vi "ExMovCollectIN.vi"() -> ()   [LabVIEW 2010]
panel:
  out "Current Wavelength":string
  in  "Increment Wavelength":dbl=50.0 format="%.2f"
  in  "End Wavelength":dbl=700.0 format="%.2f"
  in  "Start Wavelength":dbl format="%.2f"
  in  "Grating Speed":dbl=2000.0 min=1.0 step=1.0 format="%.2f"
  in  "Grating number":i16=1 min=1 max=100 step=1
  out "Strip":sgl[](graph)
  in  "Temperature":dbl=-10.0 format="%.2f"
  in  "Exposure":dbl min=0.0 step=0.001 format="%.3f"
  in  "stop":bool
  out "error out":errorcluster
  in  "error in (no error)":errorcluster
  # "ExMovCollectIN.vi\nCamera and Spectrometer control of the InSpectrum.  This vi will open both the camera and spectrograph.  It will then move the grating to the Start Wavelength.  Data will then be collected and displayed.  The sequence will be repeated after moving the grating by the Increment Wavelength until the End Wavelength is reached.  At that time, data collection will continue until the STOP button is hit."
  # "NOTES:\nA properly configured spectometer .ini must be present in the LabVIEW folder for spectrograph operation.\n\nConsult the Toolkit documentation for more information on how to configure this file."
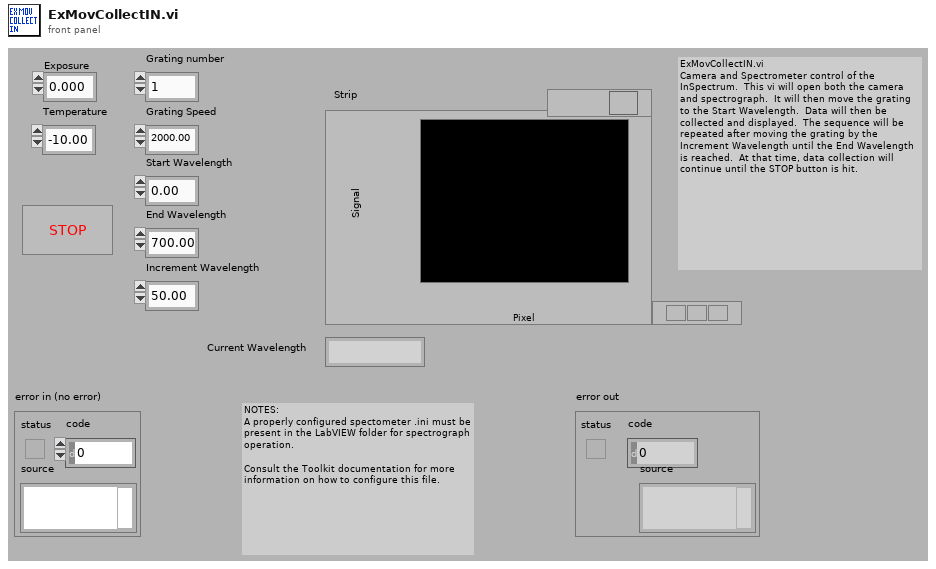
[diagram p1: front panel]
types:
  T1 = cluster{"Camera Handle":u32, "Pulser Handle":u32, "File Handle":u32, "Display Handle":u32, "Image Handle":u32}
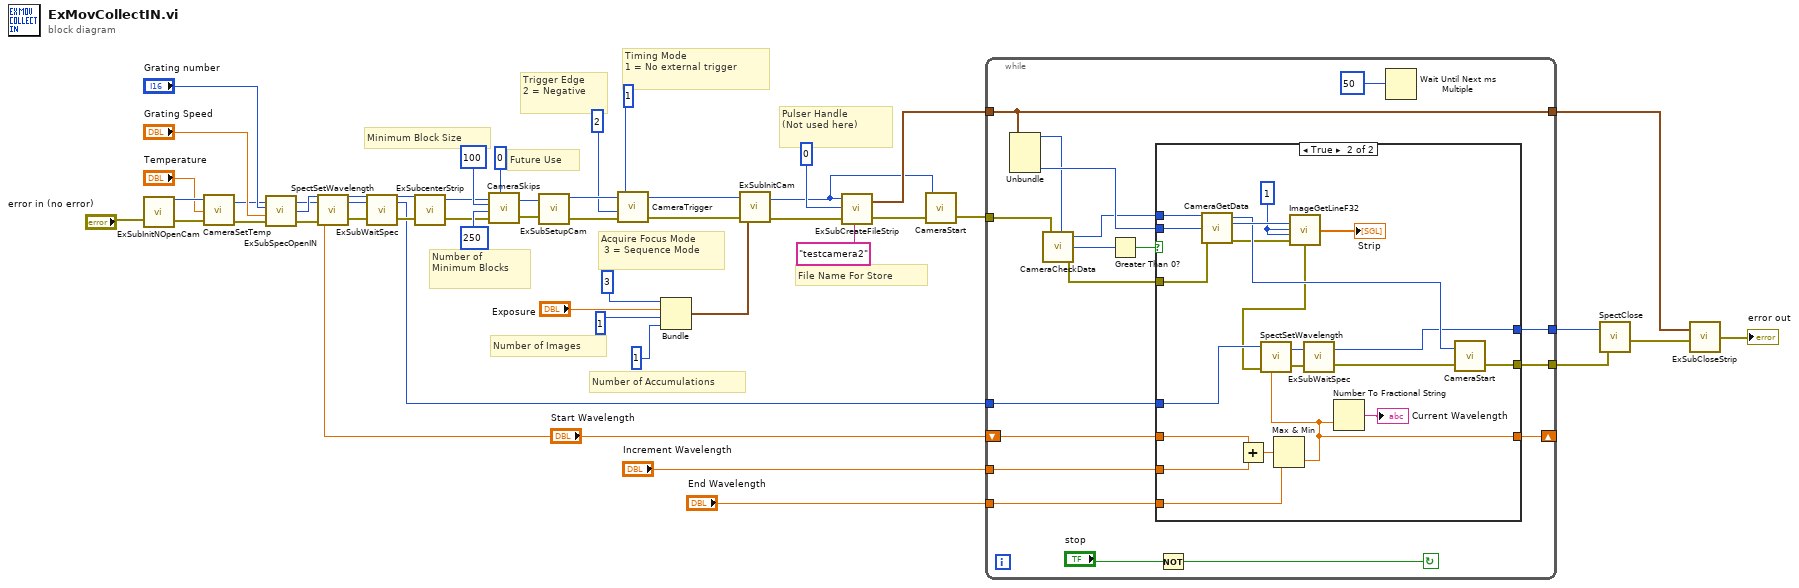
[diagram p0: block diagram]
diagram:
  # "Pulser Handle\n(Not used here)"
  # "Trigger Edge\n2 = Negative"
  # "Timing Mode\n1 = No external trigger"
  # "Future Use"
  # "Number of Minimum Blocks"
  # "Minimum Block Size"
  # "Number of Images"
  # "Number of Accumulations"
  # "Acquire Focus Mode\n 3 = Sequence Mode"
  # "File Name For Store"
  n1 = call "ExSubInitNOpenCam.vi"("error in (no error)"="error in (no error)") -> ("Camera Handle"=w4:u32, "error out"=w5:errorcluster)
  n2 = call <userlib>:"CameraSetTemp.vi"("error in (no error)"=w5, "Temperature"="Temperature", "Camera Handle"=w4) -> ("error out"=w2:errorcluster, "Camera Handle"=w3:u32)
  n3 = call "ExSubSpecOpenIN.vi"("error in (no error)"=w2, "Grating speed"="Grating Speed", "Grating number"="Grating number", "Camera Handles"=w3) -> ("error out"=w12:errorcluster, "Camera Handle"=w20:u32, "Spectrometer Handle"=w11:u32)
  n4 = call <userlib>:"SpectSetWavelength.vi"("error in"=w12, "Wavelength"="Start Wavelength", "Spectrometer Handle"=w11) -> ("error out"=w17:errorcluster, "Spectrumeter Handle"=w15:u32)
  n5 = call "ExSubWaitSpec.vi"("error in (no error)"=w17, "Spectrometer Handle"=w15) -> ("error out"=w16:errorcluster, "Spectrometer handle"=w14:u32)
  n6 = call "ExSubcenterStrip.vi"("error in (no error)"=w16, "Camera Handle"=w20) -> ("error out"=w21:errorcluster, "Camera Handle"=w22:u32)
  n7 = call <userlib>:"CameraSkips.vi"("Camera Handle"=w22, "Minimum Block Size"=100, "Number of Minimum blocks"=250, "error in"=w21, "Type of Skips"=0) -> ("Camera Handle"=w25:u32, "error out"=w24:errorcluster)
  n8 = call "ExSubSetupCam.vi"("error in (no error)"=w24, "Camera Handle"=w25) -> ("error out"=w30:errorcluster, "Camera Handle"=w34:u32)
  n9 = call <userlib>:"CameraTrigger.vi"("error in"=w30, "Trigger Edge"=2, "Timing Mode"=1, "Camera Handle"=w34) -> ("error out"=w35:errorcluster, "Camera Handle"=w33:u32)
  n10 = Bundle(3, "Exposure"="Exposure", 1, 1) -> (w42:cluster{i32, "Exposure":dbl, i32, i32})  [unwired: 1 in]
  n11 = call "ExSubInitCam.vi"("error in (no error)"=w35, "Camera Information"=w42, "Camera Handle"=w33) -> ("error out"=w41:errorcluster, "Camera Handle"=w38:u32)
  n12 = call "ExSubCreateFileStrip.vi"("error in (no error)"=w41, "File and Display Name"="testcamera2", "Pulser Handle"=0, "Camera Handle"=w38) -> ("error out"=w23:errorcluster, "Handles Out"=w39:T1)
  n13 = call <userlib>:"CameraStart.vi"("error in"=w23, "Camera Handle"=w38) -> ("error out"=w26:errorcluster)  [unwired: 1 out]
  n14 = while {
    tunnel: w39 -> [w63]
    tunnel: w26 -> [w62]
    tunnel: [w60] -> w6
    tunnel: [w63] -> w37
    tunnel: w14 -> [w54]
    tunnel: "Increment Wavelength" -> [w53]
    tunnel: "End Wavelength" -> [w52]
    shift-right: [w50] -> _
    shift-left: "Start Wavelength" -> [w51]
    tunnel: [w49] -> w7
    stop <- w64 continue-if-true
    n15 = Unbundle(w63) -> ("Camera Handle"=w58:u32, "Image Handle"=w59:u32)  [unwired: 3 out]
    n16 = call <userlib>:"CameraCheckData.vi"("Camera Handle"=w58, "error in"=w62) -> ("Camera Handle"=w57:u32, "Number Of Frames Available"=w55:i32, "error out"=w61:errorcluster)
    n17 = Greater Than 0?(x=w55) -> (x > 0?=w56:bool)
    n18 = case shown="True" w56 {
      tunnel: w61 -> [w69 w89]
      tunnel: [w69 w77] -> w60
      tunnel: w59 -> [_ w86]
      tunnel: w57 -> [_ w85]
      tunnel: w54 -> [w67 w81]
      tunnel: w53 -> [_ w74]
      tunnel: w52 -> [_ w80]
      tunnel: w51 -> [w68 w73]
      tunnel: [w68 w72] -> w50
      tunnel: [w67 w71] -> w49
      frame False {
      }
      frame True {
        w87 = 1
        n19 = call <userlib>:"CameraGetData.vi"("error in"=w89, "Data Handle"=w86, "Camera Handle"=w85) -> ("error out"=w78:errorcluster, "Data Handle"=w88:u32, "Camera Handle"=w84:u32)
        n20 = Add(x=w73, y=w74) -> (x+y=w79:dbl)
        n21 = Max & Min(x=w79, y=w80) -> (min(x,y)=w72:dbl)  [unwired: 1 out]
        n22 = call <userlib>:"ImageGetLineF32.vi"("error in"=w78, "Z Position"=w87, "Y Position"=w87, "Data Handle"=w88) -> ("error out"=w75:errorcluster, "Array F32"=→"Strip":sgl[])  [unwired: 1 out]
        n23 = call <userlib>:"SpectSetWavelength.vi"("error in"=w75, "Wavelength"=w72, "Spectrometer Handle"=w81) -> ("error out"=w83:errorcluster, "Spectrumeter Handle"=w82:u32)
        n24 = call "ExSubWaitSpec.vi"("error in (no error)"=w83, "Spectrometer Handle"=w82) -> ("error out"=w70:errorcluster, "Spectrometer handle"=w71:u32)
        n25 = Number To Fractional String(number=w72) -> (F-format string=→"Current Wavelength":string)  [unwired: 3 in]
        n26 = call <userlib>:"CameraStart.vi"("error in"=w70, "Camera Handle"=w84) -> ("error out"=w77:errorcluster)  [unwired: 1 out]
      }
    }
    n27 = Not(x="stop") -> (.not. x?=w64:bool)
    n28 = Wait Until Next ms Multiple(millisecond multiple=50) -> ()  [unwired: 1 out]
  }
  n29 = call <userlib>:"SpectClose.vi"("error in"=w6, "Spectrometer Handle"=w7) -> ("error out"=w8:errorcluster)
  n30 = call "ExSubCloseStrip.vi"("error in (no error)"=w8, "Handles In"=w37) -> ("error out"=→"error out":errorcluster)
